vi "Read Sub panel prod.vi"(8 "error in (no error)":errorcluster, 11 "coffee Actor in":refnum<class "coffee Actor.lvclass">) -> (0 "error out":errorcluster, 2 "Sub panel prod":refnum<vi>, 3 "coffee Actor out":refnum<class "coffee Actor.lvclass">)   [LabVIEW 2019, in "coffee Actor.lvlib" / "coffee Actor.lvclass"]
uses:
  coffee Actor.lvclass
  coffee Actor.lvclass/coffee Actor.ctl
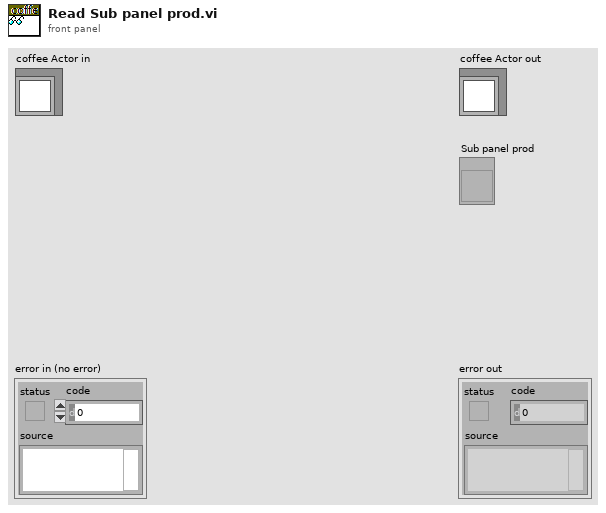
[diagram p1: front panel]
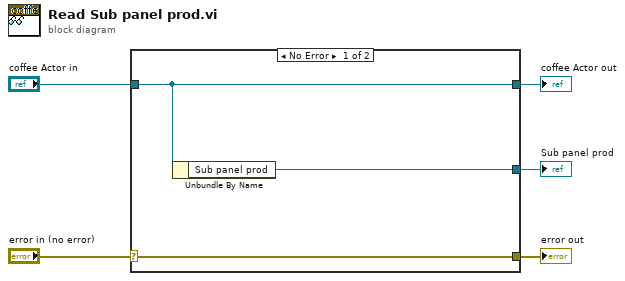
[diagram p0: block diagram]
diagram:
  n1 = case shown="No Error" "error in (no error)" {
    selector: "error in (no error)" -> [w8 w9]
    tunnel: [w8 w9] -> w4
    tunnel: [w7 w10] -> w2
    tunnel: "coffee Actor in" -> [w7 w10]
    tunnel: [w6 _] -> w1
    frame No Error {
      n2 = Unbundle By Name(w7) -> ("Sub panel prod"=w6:refnum<vi>)
    }
    frame Error {
    }
  }
  "error out" <- w4
  "coffee Actor out" <- w2
  "Sub panel prod" <- w1
